vi "Abstract LV Class - Hierarchy.vi"   [LabVIEW 2021]
uses:
  Type/Abs_Type.lvclass
  Value/Abs_Value.lvclass
  Numeric/Abs_Numeric.lvclass
  Floating Point/Abs_Floating Point.lvclass
  Single Float/Abs_Single Float.lvclass
  Double Float/Abs_Double Float.lvclass
  Extended Float/Abs_Extended Float.lvclass
  Complex Double Float/Abs_Complex Double Float.lvclass
  Complex Extended Float/Abs_Complex Extended Float.lvclass
  Complex Single Float/Abs_Complex Single Float.lvclass
  Integer/Abs_Integer.lvclass
  I8 Integer/Abs_I8 Integer.lvclass
  I16 Integer/Abs_I16 Integer.lvclass
  I32 Integer/Abs_I32 Integer.lvclass
  I64 Integer/Abs_I64 Integer.lvclass
  U8 Integer/Abs_U8 Integer.lvclass
  U16 Integer/Abs_U16 Integer.lvclass
  U32 Integer/Abs_U32 Integer.lvclass
  U64 Integer/Abs_U64 Integer.lvclass
  Time/Abs_Time.lvclass
  Boolean/Abs_Boolean.lvclass
  String/Abs_String.lvclass
  Variant/Abs_Variant.lvclass
  Waveform/Abs_Waveform.lvclass
  Boolean/Static Write.vi
  Double Float/Simple Read.vi
  Boolean/Static Read.vi
  Numeric 1D/Abs_Numeric_1D.lvclass
  Single Float 1D/Abs_Single Float 1D.lvclass
  Double Float 1D/Abs_Double Float 1D.lvclass
  Extended Float 1D/Abs_Extended Float 1D.lvclass
  Complex Double Float 1D/Abs_Complex Double Float 1D.lvclass
  Complex Extended Float 1D/Abs_Complex Extended Float 1D.lvclass
  Complex Single Float 1D/Abs_Complex Single Float 1D.lvclass
panel:
  # "SEE DIAGRAM\nFOR Hierarchy"
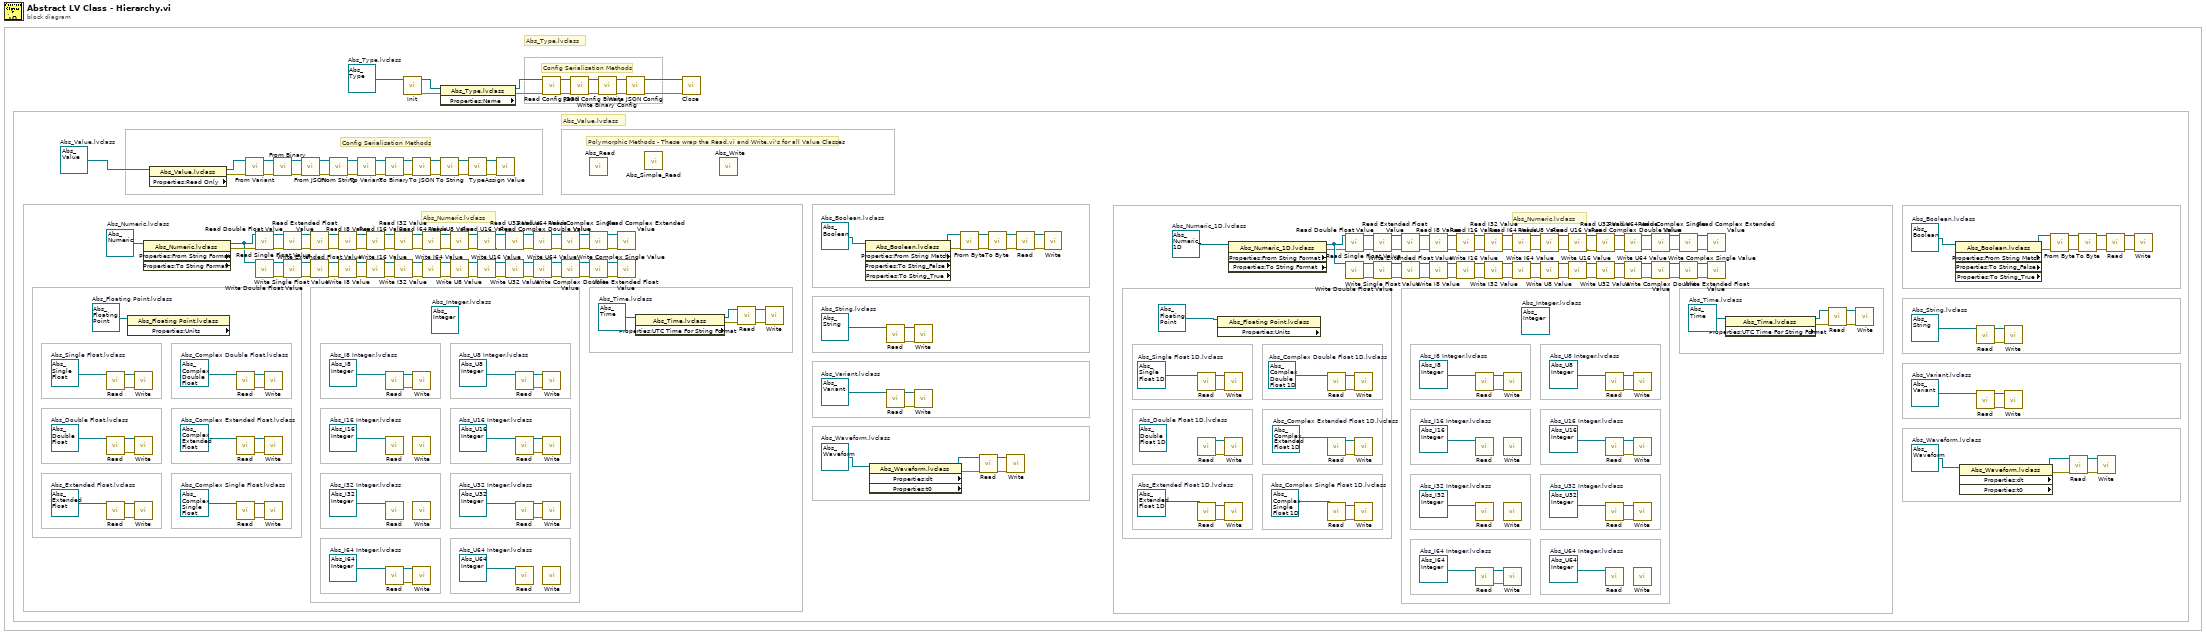
[diagram p0: block diagram]
diagram:
  w1 = refnum<class "Abs_Complex Single Float 1D.lvclass"> refnum  # Abs_Complex Single Float 1D.lvclass
  w2 = refnum<class "Abs_Complex Extended Float 1D.lvclass"> refnum  # Abs_Complex Extended Float 1D.lvclass
  w3 = refnum<class "Abs_Complex Double Float 1D.lvclass"> refnum  # Abs_Complex Double Float 1D.lvclass
  w4 = refnum<class "Abs_Extended Float 1D.lvclass"> refnum  # Abs_Extended Float 1D.lvclass
  (unwired) refnum<class "Abs_Double Float 1D.lvclass"> refnum  # Abs_Double Float 1D.lvclass
  w6 = refnum<class "Abs_Single Float 1D.lvclass"> refnum  # Abs_Single Float 1D.lvclass
  w7 = refnum<class "Abs_Numeric_1D.lvclass"> refnum  # Abs_Numeric_1D.lvclass
  w86 = refnum<class "Abs_Waveform.lvclass"> refnum  # Abs_Waveform.lvclass
  w85 = refnum<class "Abs_Variant.lvclass"> refnum  # Abs_Variant.lvclass
  w80 = refnum<class "Abs_String.lvclass"> refnum  # Abs_String.lvclass
  w71 = refnum<class "Abs_Boolean.lvclass"> refnum  # Abs_Boolean.lvclass
  w66 = refnum<class "Abs_Time.lvclass"> refnum  # Abs_Time.lvclass
  w56 = refnum<class "Abs_U64 Integer.lvclass"> refnum  # Abs_U64 Integer.lvclass
  w57 = refnum<class "Abs_U32 Integer.lvclass"> refnum  # Abs_U32 Integer.lvclass
  w59 = refnum<class "Abs_U16 Integer.lvclass"> refnum  # Abs_U16 Integer.lvclass
  w58 = refnum<class "Abs_U8 Integer.lvclass"> refnum  # Abs_U8 Integer.lvclass
  w53 = refnum<class "Abs_I64 Integer.lvclass"> refnum  # Abs_I64 Integer.lvclass
  w54 = refnum<class "Abs_I32 Integer.lvclass"> refnum  # Abs_I32 Integer.lvclass
  w55 = refnum<class "Abs_I16 Integer.lvclass"> refnum  # Abs_I16 Integer.lvclass
  w48 = refnum<class "Abs_I8 Integer.lvclass"> refnum  # Abs_I8 Integer.lvclass
  (unwired) refnum<class "Abs_Integer.lvclass"> refnum  # Abs_Integer.lvclass
  w160 = refnum<class "Abs_Waveform.lvclass"> refnum  # Abs_Waveform.lvclass
  w161 = refnum<class "Abs_Variant.lvclass"> refnum  # Abs_Variant.lvclass
  w166 = refnum<class "Abs_String.lvclass"> refnum  # Abs_String.lvclass
  w175 = refnum<class "Abs_Boolean.lvclass"> refnum  # Abs_Boolean.lvclass
  w180 = refnum<class "Abs_Time.lvclass"> refnum  # Abs_Time.lvclass
  w190 = refnum<class "Abs_U64 Integer.lvclass"> refnum  # Abs_U64 Integer.lvclass
  w189 = refnum<class "Abs_U32 Integer.lvclass"> refnum  # Abs_U32 Integer.lvclass
  w187 = refnum<class "Abs_U16 Integer.lvclass"> refnum  # Abs_U16 Integer.lvclass
  w188 = refnum<class "Abs_U8 Integer.lvclass"> refnum  # Abs_U8 Integer.lvclass
  w193 = refnum<class "Abs_I64 Integer.lvclass"> refnum  # Abs_I64 Integer.lvclass
  w192 = refnum<class "Abs_I32 Integer.lvclass"> refnum  # Abs_I32 Integer.lvclass
  w191 = refnum<class "Abs_I16 Integer.lvclass"> refnum  # Abs_I16 Integer.lvclass
  w198 = refnum<class "Abs_I8 Integer.lvclass"> refnum  # Abs_I8 Integer.lvclass
  (unwired) refnum<class "Abs_Integer.lvclass"> refnum  # Abs_Integer.lvclass
  w201 = refnum<class "Abs_Complex Single Float.lvclass"> refnum  # Abs_Complex Single Float.lvclass
  w204 = refnum<class "Abs_Complex Extended Float.lvclass"> refnum  # Abs_Complex Extended Float.lvclass
  w207 = refnum<class "Abs_Complex Double Float.lvclass"> refnum  # Abs_Complex Double Float.lvclass
  w210 = refnum<class "Abs_Extended Float.lvclass"> refnum  # Abs_Extended Float.lvclass
  w213 = refnum<class "Abs_Double Float.lvclass"> refnum  # Abs_Double Float.lvclass
  w216 = refnum<class "Abs_Single Float.lvclass"> refnum  # Abs_Single Float.lvclass
  w217 = refnum<class "Abs_Floating Point.lvclass"> refnum  # Abs_Floating Point.lvclass
  w245 = refnum<class "Abs_Numeric.lvclass"> refnum  # Abs_Numeric.lvclass
  w155 = refnum<class "Abs_Value.lvclass"> refnum  # Abs_Value.lvclass
  w268 = refnum<class "Abs_Type.lvclass"> refnum  # Abs_Type.lvclass
  # "Abs_Numeric.lvclass"
  # "Abs_Numeric.lvclass"
  # "Polymorphic Methods - These wrap the Read.vi and Write.vi's for all Value Classes"
  # "Config Serialisation Methods"
  # "Abs_Value.lvclass"
  # "Abs_Type.lvclass"
  # "Config Serialisation Methods"
  n1 = call-dynamic "Read.vi"("Double Float.lvclass_340760 in"=w216) -> ("error out"=w214:errorcluster, "Double Float.lvclass_340760 out"=w215:refnum<class "Abs_Single Float.lvclass">)  [unwired: 8 in, 1 out]
  n2 = call-dynamic "Read.vi"("Double Float.lvclass_340760 in"=w213) -> ("error out"=w211:errorcluster, "Double Float.lvclass_340760 out"=w212:refnum<class "Abs_Double Float.lvclass">)  [unwired: 8 in, 1 out]
  n3 = call-dynamic "Read.vi"("Double Float.lvclass_340760 in"=w210) -> ("error out"=w208:errorcluster, "Double Float.lvclass_340760 out"=w209:refnum<class "Abs_Extended Float.lvclass">)  [unwired: 8 in, 1 out]
  n4 = property class="Abs_Floating Point.lvclass" props=["Properties:Units"](reference=w217) -> ()  [unwired: 1 in, 3 out]
  n5 = call-dynamic "Write.vi"("error in (no error)"=w214, "Double Float.lvclass_340760 in"=w215) -> ()  [unwired: 8 in, 2 out]
  n6 = call-dynamic "Write.vi"("error in (no error)"=w211, "Double Float.lvclass in"=w212) -> ()  [unwired: 8 in, 2 out]
  n7 = call-dynamic "Write.vi"("error in (no error)"=w208, "Double Float.lvclass_340760 in"=w209) -> ()  [unwired: 8 in, 2 out]
  n8 = property class="Abs_Numeric.lvclass" props=["Properties:From String Format", "Properties:To String Format"](reference=w245) -> (reference out=w146:refnum<class "Abs_Numeric.lvclass">, error out=w244:errorcluster)  [unwired: 1 in, 2 out]
  n9 = property class="Abs_Value.lvclass" props=["Properties:Read Only"](reference=w155) -> (reference out=w153:refnum<class "Abs_Value.lvclass">, error out=w154:errorcluster)  [unwired: 1 in, 1 out]
  n10 = call-dynamic "Read.vi"("Double Float.lvclass_340760 in"=w207) -> ("error out"=w205:errorcluster, "Double Float.lvclass_340760 out"=w206:refnum<class "Abs_Complex Double Float.lvclass">)  [unwired: 8 in, 1 out]
  n11 = call-dynamic "Read.vi"("Double Float.lvclass_340760 in"=w204) -> ("error out"=w202:errorcluster, "Double Float.lvclass_340760 out"=w203:refnum<class "Abs_Complex Extended Float.lvclass">)  [unwired: 8 in, 1 out]
  n12 = call-dynamic "Read.vi"("Double Float.lvclass_340760 in"=w201) -> ("error out"=w199:errorcluster, "Double Float.lvclass_340760 out"=w200:refnum<class "Abs_Complex Single Float.lvclass">)  [unwired: 8 in, 1 out]
  n13 = call-dynamic "From Variant.vi"("error in (no error)"=w154, "Abs_Value in"=w153) -> ("error out"=w151:errorcluster, "Abs_Value out"=w152:refnum<class "Abs_Value.lvclass">)  [unwired: 8 in]
  n14 = call-dynamic "Read Double Float Value.vi"("error in (no error)"=w244, "Numeric in"=w146) -> ("error out"=w234:errorcluster, "Numeric out"=w243:refnum<class "Abs_Numeric.lvclass">)  [unwired: 7 in, 1 out]
  n15 = call-dynamic "Write Double Float Value.vi"("Numeric in"=w146) -> ("error out"=w132:errorcluster, "Numeric out"=w145:refnum<class "Abs_Numeric.lvclass">)  [unwired: 9 in]
  n16 = call-dynamic "Write.vi"("error in (no error)"=w205, "Double Float.lvclass_340760 in"=w206) -> ()  [unwired: 8 in, 2 out]
  n17 = call-dynamic "Write.vi"("error in (no error)"=w202, "Double Float.lvclass_340760 in"=w203) -> ()  [unwired: 8 in, 2 out]
  n18 = call-dynamic "Write.vi"("error in (no error)"=w199, "Double Float.lvclass_340760 in"=w200) -> ()  [unwired: 8 in, 2 out]
  n19 = call-dynamic "From Binary.vi"("error in (no error)"=w151, "Type in"=w152) -> ("error out"=w250:errorcluster, "Type out"=w255:refnum<class "Abs_Value.lvclass">)  [unwired: 7 in, 1 out]
  n20 = call-dynamic "Read Single Float Value.vi"("error in (no error)"=w234, "Numeric in"=w243) -> ("error out"=w233:errorcluster, "Numeric out"=w242:refnum<class "Abs_Numeric.lvclass">)  [unwired: 7 in, 1 out]
  n21 = call-dynamic "Write Single Float Value.vi"("error in (no error)"=w132, "Numeric in"=w145) -> ("error out"=w131:errorcluster, "Numeric out"=w144:refnum<class "Abs_Numeric.lvclass">)  [unwired: 8 in]
  n22 = call-dynamic "From JSON.vi"("error in (no error)"=w250, "Type in"=w255) -> ("error out"=w249:errorcluster, "Type out"=w254:refnum<class "Abs_Value.lvclass">)  [unwired: 8 in]
  n23 = call-dynamic "Read Extended Float Value.vi"("error in (no error)"=w233, "Numeric in"=w242) -> ("error out"=w232:errorcluster, "Numeric out"=w241:refnum<class "Abs_Numeric.lvclass">)  [unwired: 7 in, 1 out]
  n24 = call-dynamic "Write Extended Float Value.vi"("error in (no error)"=w131, "Numeric in"=w144) -> ("error out"=w130:errorcluster, "Numeric out"=w143:refnum<class "Abs_Numeric.lvclass">)  [unwired: 8 in]
  n25 = call-dynamic "From String.vi"("error in (no error)"=w249, "Type in"=w254) -> ("error out"=w149:errorcluster, "Type out"=w150:refnum<class "Abs_Value.lvclass">)  [unwired: 6 in, 2 out]
  n26 = call-dynamic "Read I8 Value.vi"("error in (no error)"=w232, "Numeric in"=w241) -> ("error out"=w231:errorcluster, "Numeric out"=w240:refnum<class "Abs_Numeric.lvclass">)  [unwired: 7 in, 1 out]
  n27 = call-dynamic "Write I8 Value.vi"("error in (no error)"=w130, "Numeric in"=w143) -> ("error out"=w129:errorcluster, "Numeric out"=w142:refnum<class "Abs_Numeric.lvclass">)  [unwired: 8 in]
  n28 = call-dynamic "To Variant.vi"("error in (no error)"=w149, "Abs_Value in"=w150) -> ("error out"=w147:errorcluster, "Abs_Value out"=w148:refnum<class "Abs_Value.lvclass">)  [unwired: 7 in, 1 out]
  n29 = call-dynamic "Read I16 Value.vi"("error in (no error)"=w231, "Numeric in"=w240) -> ("error out"=w230:errorcluster, "Numeric out"=w239:refnum<class "Abs_Numeric.lvclass">)  [unwired: 7 in, 1 out]
  n30 = call-dynamic "Write I16 Value.vi"("error in (no error)"=w129, "Numeric in"=w142) -> ("error out"=w128:errorcluster, "Numeric out"=w141:refnum<class "Abs_Numeric.lvclass">)  [unwired: 8 in]
  n31 = call-dynamic "To Binary.vi"("error in (no error)"=w147, "Type in"=w148) -> ("error out"=w248:errorcluster, "Type out"=w253:refnum<class "Abs_Value.lvclass">)  [unwired: 7 in, 1 out]
  n32 = call-dynamic "Read.vi"("Double Float.lvclass_340760 in"=w198) -> ("error out"=w196:errorcluster, "Double Float.lvclass_340760 out"=w197:refnum<class "Abs_I8 Integer.lvclass">)  [unwired: 8 in, 1 out]
  n33 = call-dynamic "Read.vi"("Double Float.lvclass_340760 in"=w191) -> ()  [unwired: 8 in, 3 out]
  n34 = call-dynamic "Read.vi"("Double Float.lvclass_340760 in"=w192) -> ()  [unwired: 8 in, 3 out]
  n35 = call-dynamic "Read.vi"("Double Float.lvclass_340760 in"=w193) -> ("error out"=w194:errorcluster, "Double Float.lvclass_340760 out"=w195:refnum<class "Abs_I64 Integer.lvclass">)  [unwired: 8 in, 1 out]
  n36 = call-dynamic "Read I32 Value.vi"("error in (no error)"=w230, "Numeric in"=w239) -> ("error out"=w229:errorcluster, "Numeric out"=w238:refnum<class "Abs_Numeric.lvclass">)  [unwired: 7 in, 1 out]
  n37 = call-dynamic "Write I32 Value.vi"("error in (no error)"=w128, "Numeric in"=w141) -> ("error out"=w127:errorcluster, "Numeric out"=w140:refnum<class "Abs_Numeric.lvclass">)  [unwired: 8 in]
  n38 = call-dynamic "Init.vi"("Data in"=w268) -> ("error out"=w267:errorcluster, "Data out"=w266:refnum<class "Abs_Type.lvclass">)  [unwired: 9 in]
  n39 = call-dynamic "To JSON.vi"("error in (no error)"=w248, "Type in"=w253) -> ("error out"=w247:errorcluster, "Type out"=w252:refnum<class "Abs_Value.lvclass">)  [unwired: 7 in, 1 out]
  n40 = call-dynamic "Write.vi"("error in (no error)"=w196, "Double Float.lvclass_340760 in"=w197) -> ()  [unwired: 8 in, 2 out]
  n41 = call-dynamic "Write.vi"() -> ()  [unwired: 10 in, 2 out]
  n42 = call-dynamic "Write.vi"() -> ()  [unwired: 10 in, 2 out]
  n43 = call-dynamic "Write.vi"("error in (no error)"=w194, "Double Float.lvclass_340760 in"=w195) -> ()  [unwired: 8 in, 2 out]
  n44 = call-dynamic "Read I64 Value.vi"("error in (no error)"=w229, "Numeric in"=w238) -> ("error out"=w228:errorcluster, "Numeric out"=w237:refnum<class "Abs_Numeric.lvclass">)  [unwired: 7 in, 1 out]
  n45 = call-dynamic "Write I64 Value.vi"("error in (no error)"=w127, "Numeric in"=w140) -> ("error out"=w126:errorcluster, "Numeric out"=w139:refnum<class "Abs_Numeric.lvclass">)  [unwired: 8 in]
  n46 = property class="Abs_Type.lvclass" props=["Properties:Name"](reference=w266, error in=w267) -> (reference out=w264:refnum<class "Abs_Type.lvclass">, error out=w265:errorcluster)  [unwired: 1 out]
  n47 = call-dynamic "To String.vi"("error in (no error)"=w247, "Types in"=w252) -> ("error out"=w246:errorcluster, "Types out"=w251:refnum<class "Abs_Value.lvclass">)  [unwired: 7 in, 1 out]
  n48 = call-dynamic "Read U8 Value.vi"("error in (no error)"=w228, "Numeric in"=w237) -> ("error out"=w227:errorcluster, "Numeric out"=w236:refnum<class "Abs_Numeric.lvclass">)  [unwired: 7 in, 1 out]
  n49 = call-dynamic "Write U8 Value.vi"("error in (no error)"=w126, "Numeric in"=w139) -> ("error out"=w125:errorcluster, "Numeric out"=w138:refnum<class "Abs_Numeric.lvclass">)  [unwired: 8 in]
  n50 = call-dynamic "Type.vi"("error in (no error)"=w246, "Element in"=w251) -> ("error out"=w118:errorcluster, "Element out"=w119:refnum<class "Abs_Value.lvclass">)  [unwired: 7 in, 1 out]
  n51 = call-dynamic "Read U16 Value.vi"("error in (no error)"=w227, "Numeric in"=w236) -> ("error out"=w226:errorcluster, "Numeric out"=w235:refnum<class "Abs_Numeric.lvclass">)  [unwired: 7 in, 1 out]
  n52 = call-dynamic "Write U16 Value.vi"("error in (no error)"=w125, "Numeric in"=w138) -> ("error out"=w124:errorcluster, "Numeric out"=w137:refnum<class "Abs_Numeric.lvclass">)  [unwired: 8 in]
  n53 = call-dynamic "Assign Value.vi"("error in (no error)"=w118, "Abs_Value in"=w119) -> ()  [unwired: 8 in, 2 out]
  n54 = call-dynamic "Read U32 Value.vi"("error in (no error)"=w226, "Numeric in"=w235) -> ("error out"=w225:errorcluster, "Numeric out"=w224:refnum<class "Abs_Numeric.lvclass">)  [unwired: 7 in, 1 out]
  n55 = call-dynamic "Write U32 Value.vi"("error in (no error)"=w124, "Numeric in"=w137) -> ("error out"=w123:errorcluster, "Numeric out"=w136:refnum<class "Abs_Numeric.lvclass">)  [unwired: 8 in]
  n56 = call-dynamic "Read.vi"("Double Float.lvclass_340760 in"=w188) -> ("error out"=w185:errorcluster, "Double Float.lvclass_340760 out"=w186:refnum<class "Abs_U8 Integer.lvclass">)  [unwired: 8 in, 1 out]
  n57 = call-dynamic "Read.vi"("Double Float.lvclass_340760 in"=w187) -> ("error out"=w183:errorcluster, "Double Float.lvclass_340760 out"=w184:refnum<class "Abs_U16 Integer.lvclass">)  [unwired: 8 in, 1 out]
  n58 = call-dynamic "Read.vi"("Double Float.lvclass_340760 in"=w189) -> ("error out"=w181:errorcluster, "Double Float.lvclass_340760 out"=w182:refnum<class "Abs_U32 Integer.lvclass">)  [unwired: 8 in, 1 out]
  n59 = call-dynamic "Read.vi"("Double Float.lvclass_340760 in"=w190) -> ()  [unwired: 8 in, 3 out]
  n60 = call-dynamic "Read U64 Value.vi"("error in (no error)"=w225, "Numeric in"=w224) -> ("error out"=w222:errorcluster, "Numeric out"=w223:refnum<class "Abs_Numeric.lvclass">)  [unwired: 7 in, 1 out]
  n61 = call-dynamic "Write U64 Value.vi"("error in (no error)"=w123, "Numeric in"=w136) -> ("error out"=w122:errorcluster, "Numeric out"=w135:refnum<class "Abs_Numeric.lvclass">)  [unwired: 8 in]
  n62 = call "Read Config JSON.vi"("error in (no error)"=w265, "Abs_Type in"=w264) -> ("error out"=w263:errorcluster, "Abs_Type out"=w262:refnum<class "Abs_Type.lvclass">)  [unwired: 8 in]
  n63 = call-dynamic "Write.vi"("error in (no error)"=w185, "Double Float.lvclass_340760 in"=w186) -> ()  [unwired: 8 in, 2 out]
  n64 = call-dynamic "Write.vi"("error in (no error)"=w183, "Double Float.lvclass_340760 in"=w184) -> ()  [unwired: 8 in, 2 out]
  n65 = call-dynamic "Write.vi"("error in (no error)"=w181, "Double Float.lvclass_340760 in"=w182) -> ()  [unwired: 8 in, 2 out]
  n66 = call-dynamic "Write.vi"() -> ()  [unwired: 10 in, 2 out]
  n67 = call-dynamic "Read Complex Double Value.vi"("error in (no error)"=w222, "Numeric in"=w223) -> ("error out"=w221:errorcluster, "Numeric out"=w220:refnum<class "Abs_Numeric.lvclass">)  [unwired: 7 in, 1 out]
  n68 = call-dynamic "Write Complex Double Value.vi"("error in (no error)"=w122, "Numeric in"=w135) -> ("error out"=w121:errorcluster, "Numeric out"=w134:refnum<class "Abs_Numeric.lvclass">)  [unwired: 8 in]
  n69 = call "Read Config Binary.vi"("error in (no error)"=w263, "Abs_Type in"=w262) -> ("error out"=w261:errorcluster, "Abs_Type out"=w260:refnum<class "Abs_Type.lvclass">)  [unwired: 7 in, 1 out]
  n70 = call-poly "Abs_Read.vi"() -> ()  [unwired: 9 in, 3 out]
  n71 = call-dynamic "Read Complex Single Value.vi"("error in (no error)"=w221, "Numeric in"=w220) -> ("error out"=w218:errorcluster, "Numeric out"=w219:refnum<class "Abs_Numeric.lvclass">)  [unwired: 7 in, 1 out]
  n72 = call-dynamic "Write Complex Single Value.vi"("error in (no error)"=w121, "Numeric in"=w134) -> ("error out"=w120:errorcluster, "Numeric out"=w133:refnum<class "Abs_Numeric.lvclass">)  [unwired: 8 in]
  n73 = call-dynamic "Write Binary Config.vi"("error in (no error)"=w261, "Abs_Type in"=w260) -> ("error out"=w258:errorcluster, "Abs_Type out"=w259:refnum<class "Abs_Type.lvclass">)  [unwired: 7 in, 1 out]
  n74 = call-dynamic "Read Complex Extended Value.vi"("error in (no error)"=w218, "Numeric in"=w219) -> ()  [unwired: 7 in, 3 out]
  n75 = call-dynamic "Write Extended Float Value.vi"("error in (no error)"=w120, "Numeric in"=w133) -> ()  [unwired: 8 in, 2 out]
  n76 = call-dynamic "Write JSON Config.vi"("error in (no error)"=w258, "Abs_Type in"=w259) -> ("error out"=w257:errorcluster, "Abs_Type out"=w256:refnum<class "Abs_Type.lvclass">)  [unwired: 7 in, 1 out]
  n77 = property class="Abs_Time.lvclass" props=["Properties:UTC Time For String Format"](reference=w180) -> (reference out=w176:refnum<class "Abs_Time.lvclass">, error out=w179:errorcluster)  [unwired: 1 in, 1 out]
  n78 = call-poly "Abs_Simple_Read.vi"() -> ()  [unwired: 5 in, 1 out]
  n79 = call-dynamic "Close.vi"("error in (no error)"=w257, "Data in"=w256) -> ()  [unwired: 8 in, 2 out]
  n80 = call-poly "Abs_Write.vi"() -> ()  [unwired: 10 in, 2 out]
  n81 = call-dynamic "Read.vi"("error in (no error)"=w179, "Double Float.lvclass_340760 in"=w176) -> ("error out"=w178:errorcluster, "Double Float.lvclass_340760 out"=w177:refnum<class "Abs_Time.lvclass">)  [unwired: 7 in, 1 out]
  n82 = call-dynamic "Write.vi"("error in (no error)"=w178, "Double Float.lvclass_340760 in"=w177) -> ()  [unwired: 8 in, 2 out]
  n83 = property class="Abs_Boolean.lvclass" props=["Properties:From String Match", "Properties:To String_False", "Properties:To String_True"](reference=w175) -> (reference out=w173:refnum<class "Abs_Boolean.lvclass">, error out=w174:errorcluster)  [unwired: 1 in, 3 out]
  n84 = property class="Abs_Waveform.lvclass" props=["Properties:dt", "Properties:t0"](reference=w160) -> (reference out=w159:refnum<class "Abs_Waveform.lvclass">, error out=w158:errorcluster)  [unwired: 1 in, 2 out]
  n85 = call-dynamic "Read.vi"("Abs_String in"=w166) -> ("error out"=w164:errorcluster, "Abs_String out"=w165:refnum<class "Abs_String.lvclass">)  [unwired: 8 in, 1 out]
  n86 = call-dynamic "Read.vi"("Abs_Variant in"=w161) -> ("error out"=w162:errorcluster, "Abs_Variant out"=w163:refnum<class "Abs_Variant.lvclass">)  [unwired: 8 in, 1 out]
  n87 = call-dynamic "Write.vi"("error in (no error)"=w164, "Abs_String in"=w165) -> ()  [unwired: 8 in, 2 out]
  n88 = call-dynamic "Write.vi"("error in (no error)"=w162, "Abs_Variant in"=w163) -> ()  [unwired: 8 in, 2 out]
  n89 = call-dynamic "From Byte.vi"("error in (no error)"=w174, "Boolean in"=w173) -> ("error out"=w171:errorcluster, "Boolean out"=w172:refnum<class "Abs_Boolean.lvclass">)  [unwired: 8 in]
  n90 = call-dynamic "Read.vi"("error in (no error)"=w158, "Abs_Waveform in"=w159) -> ("error out"=w157:errorcluster, "Abs_Waveform out"=w156:refnum<class "Abs_Waveform.lvclass">)  [unwired: 7 in, 1 out]
  n91 = call-dynamic "To Byte.vi"("error in (no error)"=w171, "Boolean in"=w172) -> ("error out"=w169:errorcluster, "Boolean out"=w170:refnum<class "Abs_Boolean.lvclass">)  [unwired: 8 in]
  n92 = call-dynamic "Write.vi"("error in (no error)"=w157, "Abs_Waveform in"=w156) -> ()  [unwired: 8 in, 2 out]
  n93 = call-dynamic "Read.vi"("error in (no error)"=w169, "Boolean in"=w170) -> ("error out"=w167:errorcluster, "Boolean out"=w168:refnum<class "Abs_Boolean.lvclass">)  [unwired: 7 in, 1 out]
  n94 = call-dynamic "Write.vi"("error in (no error)"=w167, "Boolean in"=w168) -> ()  [unwired: 8 in, 2 out]
  n95 = call-dynamic "Read.vi"("Double Float.lvclass_340760 in"=w6) -> ("error out"=w36:errorcluster, "Double Float.lvclass_340760 out"=w35:refnum<class "Abs_Single Float.lvclass">)  [unwired: 8 in, 1 out]
  n96 = call-dynamic "Read.vi"() -> ("error out"=w39:errorcluster, "Double Float.lvclass_340760 out"=w38:refnum<class "Abs_Double Float.lvclass">, "Double Float.lvclass_340760 in"=w37:refnum<class "Abs_Double Float.lvclass">)  [unwired: 8 in, 1 out]
  n97 = call-dynamic "Read.vi"("Double Float.lvclass_340760 in"=w4) -> ("error out"=w41:errorcluster, "Double Float.lvclass_340760 out"=w40:refnum<class "Abs_Extended Float.lvclass">)  [unwired: 8 in, 1 out]
  n98 = property class="Abs_Floating Point.lvclass" props=["Properties:Units"](reference=refnum<class "Abs_Floating Point.lvclass"> refnum ("Abs_Floating Point.lvclass")) -> ()  [unwired: 1 in, 3 out]
  n99 = call-dynamic "Write.vi"("error in (no error)"=w36, "Double Float.lvclass_340760 in"=w35) -> ()  [unwired: 8 in, 2 out]
  n100 = call-dynamic "Write.vi"("error in (no error)"=w39, "Double Float.lvclass in"=w38) -> ()  [unwired: 8 in, 2 out]
  n101 = call-dynamic "Write.vi"("error in (no error)"=w41, "Double Float.lvclass_340760 in"=w40) -> ()  [unwired: 8 in, 2 out]
  n102 = property class="Abs_Numeric_1D.lvclass" props=["Properties:From String Format", "Properties:To String Format"](reference=w7) -> (reference out=w91:refnum<class "Abs_Numeric_1D.lvclass">, error out=w8:errorcluster)  [unwired: 1 in, 2 out]
  n103 = call-dynamic "Read.vi"("Double Float.lvclass_340760 in"=w3) -> ("error out"=w43:errorcluster, "Double Float.lvclass_340760 out"=w42:refnum<class "Abs_Complex Double Float.lvclass">)  [unwired: 8 in, 1 out]
  n104 = call-dynamic "Read.vi"("Double Float.lvclass_340760 in"=w2) -> ("error out"=w45:errorcluster, "Double Float.lvclass_340760 out"=w44:refnum<class "Abs_Complex Extended Float.lvclass">)  [unwired: 8 in, 1 out]
  n105 = call-dynamic "Read.vi"("Double Float.lvclass_340760 in"=w1) -> ("error out"=w47:errorcluster, "Double Float.lvclass_340760 out"=w46:refnum<class "Abs_Complex Single Float.lvclass">)  [unwired: 8 in, 1 out]
  n106 = call-dynamic "Read Double Float Value.vi"("error in (no error)"=w8, "Numeric in"=w91) -> ("error out"=w18:errorcluster, "Numeric out"=w9:refnum<class "Abs_Numeric.lvclass">)  [unwired: 7 in, 1 out]
  n107 = call-dynamic "Write Double Float Value.vi"("Numeric in"=w91) -> ("error out"=w105:errorcluster, "Numeric out"=w92:refnum<class "Abs_Numeric.lvclass">)  [unwired: 9 in]
  n108 = call-dynamic "Write.vi"("error in (no error)"=w43, "Double Float.lvclass_340760 in"=w42) -> ()  [unwired: 8 in, 2 out]
  n109 = call-dynamic "Write.vi"("error in (no error)"=w45, "Double Float.lvclass_340760 in"=w44) -> ()  [unwired: 8 in, 2 out]
  n110 = call-dynamic "Write.vi"("error in (no error)"=w47, "Double Float.lvclass_340760 in"=w46) -> ()  [unwired: 8 in, 2 out]
  n111 = call-dynamic "Read Single Float Value.vi"("error in (no error)"=w18, "Numeric in"=w9) -> ("error out"=w19:errorcluster, "Numeric out"=w10:refnum<class "Abs_Numeric.lvclass">)  [unwired: 7 in, 1 out]
  n112 = call-dynamic "Write Single Float Value.vi"("error in (no error)"=w105, "Numeric in"=w92) -> ("error out"=w106:errorcluster, "Numeric out"=w93:refnum<class "Abs_Numeric.lvclass">)  [unwired: 8 in]
  n113 = call-dynamic "Read Extended Float Value.vi"("error in (no error)"=w19, "Numeric in"=w10) -> ("error out"=w20:errorcluster, "Numeric out"=w11:refnum<class "Abs_Numeric.lvclass">)  [unwired: 7 in, 1 out]
  n114 = call-dynamic "Write Extended Float Value.vi"("error in (no error)"=w106, "Numeric in"=w93) -> ("error out"=w107:errorcluster, "Numeric out"=w94:refnum<class "Abs_Numeric.lvclass">)  [unwired: 8 in]
  n115 = call-dynamic "Read I8 Value.vi"("error in (no error)"=w20, "Numeric in"=w11) -> ("error out"=w21:errorcluster, "Numeric out"=w12:refnum<class "Abs_Numeric.lvclass">)  [unwired: 7 in, 1 out]
  n116 = call-dynamic "Write I8 Value.vi"("error in (no error)"=w107, "Numeric in"=w94) -> ("error out"=w108:errorcluster, "Numeric out"=w95:refnum<class "Abs_Numeric.lvclass">)  [unwired: 8 in]
  n117 = call-dynamic "Read I16 Value.vi"("error in (no error)"=w21, "Numeric in"=w12) -> ("error out"=w22:errorcluster, "Numeric out"=w13:refnum<class "Abs_Numeric.lvclass">)  [unwired: 7 in, 1 out]
  n118 = call-dynamic "Write I16 Value.vi"("error in (no error)"=w108, "Numeric in"=w95) -> ("error out"=w109:errorcluster, "Numeric out"=w96:refnum<class "Abs_Numeric.lvclass">)  [unwired: 8 in]
  n119 = call-dynamic "Read.vi"("Double Float.lvclass_340760 in"=w48) -> ("error out"=w50:errorcluster, "Double Float.lvclass_340760 out"=w49:refnum<class "Abs_I8 Integer.lvclass">)  [unwired: 8 in, 1 out]
  n120 = call-dynamic "Read.vi"("Double Float.lvclass_340760 in"=w55) -> ()  [unwired: 8 in, 3 out]
  n121 = call-dynamic "Read.vi"("Double Float.lvclass_340760 in"=w54) -> ()  [unwired: 8 in, 3 out]
  n122 = call-dynamic "Read.vi"("Double Float.lvclass_340760 in"=w53) -> ("error out"=w52:errorcluster, "Double Float.lvclass_340760 out"=w51:refnum<class "Abs_I64 Integer.lvclass">)  [unwired: 8 in, 1 out]
  n123 = call-dynamic "Read I32 Value.vi"("error in (no error)"=w22, "Numeric in"=w13) -> ("error out"=w23:errorcluster, "Numeric out"=w14:refnum<class "Abs_Numeric.lvclass">)  [unwired: 7 in, 1 out]
  n124 = call-dynamic "Write I32 Value.vi"("error in (no error)"=w109, "Numeric in"=w96) -> ("error out"=w110:errorcluster, "Numeric out"=w97:refnum<class "Abs_Numeric.lvclass">)  [unwired: 8 in]
  n125 = call-dynamic "Write.vi"("error in (no error)"=w50, "Double Float.lvclass_340760 in"=w49) -> ()  [unwired: 8 in, 2 out]
  n126 = call-dynamic "Write.vi"() -> ()  [unwired: 10 in, 2 out]
  n127 = call-dynamic "Write.vi"() -> ()  [unwired: 10 in, 2 out]
  n128 = call-dynamic "Write.vi"("error in (no error)"=w52, "Double Float.lvclass_340760 in"=w51) -> ()  [unwired: 8 in, 2 out]
  n129 = call-dynamic "Read I64 Value.vi"("error in (no error)"=w23, "Numeric in"=w14) -> ("error out"=w24:errorcluster, "Numeric out"=w15:refnum<class "Abs_Numeric.lvclass">)  [unwired: 7 in, 1 out]
  n130 = call-dynamic "Write I64 Value.vi"("error in (no error)"=w110, "Numeric in"=w97) -> ("error out"=w111:errorcluster, "Numeric out"=w98:refnum<class "Abs_Numeric.lvclass">)  [unwired: 8 in]
  n131 = call-dynamic "Read U8 Value.vi"("error in (no error)"=w24, "Numeric in"=w15) -> ("error out"=w25:errorcluster, "Numeric out"=w16:refnum<class "Abs_Numeric.lvclass">)  [unwired: 7 in, 1 out]
  n132 = call-dynamic "Write U8 Value.vi"("error in (no error)"=w111, "Numeric in"=w98) -> ("error out"=w112:errorcluster, "Numeric out"=w99:refnum<class "Abs_Numeric.lvclass">)  [unwired: 8 in]
  n133 = call-dynamic "Read U16 Value.vi"("error in (no error)"=w25, "Numeric in"=w16) -> ("error out"=w26:errorcluster, "Numeric out"=w17:refnum<class "Abs_Numeric.lvclass">)  [unwired: 7 in, 1 out]
  n134 = call-dynamic "Write U16 Value.vi"("error in (no error)"=w112, "Numeric in"=w99) -> ("error out"=w113:errorcluster, "Numeric out"=w100:refnum<class "Abs_Numeric.lvclass">)  [unwired: 8 in]
  n135 = call-dynamic "Read U32 Value.vi"("error in (no error)"=w26, "Numeric in"=w17) -> ("error out"=w27:errorcluster, "Numeric out"=w28:refnum<class "Abs_Numeric.lvclass">)  [unwired: 7 in, 1 out]
  n136 = call-dynamic "Write U32 Value.vi"("error in (no error)"=w113, "Numeric in"=w100) -> ("error out"=w114:errorcluster, "Numeric out"=w101:refnum<class "Abs_Numeric.lvclass">)  [unwired: 8 in]
  n137 = call-dynamic "Read.vi"("Double Float.lvclass_340760 in"=w58) -> ("error out"=w61:errorcluster, "Double Float.lvclass_340760 out"=w60:refnum<class "Abs_U8 Integer.lvclass">)  [unwired: 8 in, 1 out]
  n138 = call-dynamic "Read.vi"("Double Float.lvclass_340760 in"=w59) -> ("error out"=w63:errorcluster, "Double Float.lvclass_340760 out"=w62:refnum<class "Abs_U16 Integer.lvclass">)  [unwired: 8 in, 1 out]
  n139 = call-dynamic "Read.vi"("Double Float.lvclass_340760 in"=w57) -> ("error out"=w65:errorcluster, "Double Float.lvclass_340760 out"=w64:refnum<class "Abs_U32 Integer.lvclass">)  [unwired: 8 in, 1 out]
  n140 = call-dynamic "Read.vi"("Double Float.lvclass_340760 in"=w56) -> ()  [unwired: 8 in, 3 out]
  n141 = call-dynamic "Read U64 Value.vi"("error in (no error)"=w27, "Numeric in"=w28) -> ("error out"=w30:errorcluster, "Numeric out"=w29:refnum<class "Abs_Numeric.lvclass">)  [unwired: 7 in, 1 out]
  n142 = call-dynamic "Write U64 Value.vi"("error in (no error)"=w114, "Numeric in"=w101) -> ("error out"=w115:errorcluster, "Numeric out"=w102:refnum<class "Abs_Numeric.lvclass">)  [unwired: 8 in]
  n143 = call-dynamic "Write.vi"("error in (no error)"=w61, "Double Float.lvclass_340760 in"=w60) -> ()  [unwired: 8 in, 2 out]
  n144 = call-dynamic "Write.vi"("error in (no error)"=w63, "Double Float.lvclass_340760 in"=w62) -> ()  [unwired: 8 in, 2 out]
  n145 = call-dynamic "Write.vi"("error in (no error)"=w65, "Double Float.lvclass_340760 in"=w64) -> ()  [unwired: 8 in, 2 out]
  n146 = call-dynamic "Write.vi"() -> ()  [unwired: 10 in, 2 out]
  n147 = call-dynamic "Read Complex Double Value.vi"("error in (no error)"=w30, "Numeric in"=w29) -> ("error out"=w31:errorcluster, "Numeric out"=w32:refnum<class "Abs_Numeric.lvclass">)  [unwired: 7 in, 1 out]
  n148 = call-dynamic "Write Complex Double Value.vi"("error in (no error)"=w115, "Numeric in"=w102) -> ("error out"=w116:errorcluster, "Numeric out"=w103:refnum<class "Abs_Numeric.lvclass">)  [unwired: 8 in]
  n149 = call-dynamic "Read Complex Single Value.vi"("error in (no error)"=w31, "Numeric in"=w32) -> ("error out"=w34:errorcluster, "Numeric out"=w33:refnum<class "Abs_Numeric.lvclass">)  [unwired: 7 in, 1 out]
  n150 = call-dynamic "Write Complex Single Value.vi"("error in (no error)"=w116, "Numeric in"=w103) -> ("error out"=w117:errorcluster, "Numeric out"=w104:refnum<class "Abs_Numeric.lvclass">)  [unwired: 8 in]
  n151 = call-dynamic "Read Complex Extended Value.vi"("error in (no error)"=w34, "Numeric in"=w33) -> ()  [unwired: 7 in, 3 out]
  n152 = call-dynamic "Write Extended Float Value.vi"("error in (no error)"=w117, "Numeric in"=w104) -> ()  [unwired: 8 in, 2 out]
  n153 = property class="Abs_Time.lvclass" props=["Properties:UTC Time For String Format"](reference=w66) -> (reference out=w70:refnum<class "Abs_Time.lvclass">, error out=w67:errorcluster)  [unwired: 1 in, 1 out]
  n154 = call-dynamic "Read.vi"("error in (no error)"=w67, "Double Float.lvclass_340760 in"=w70) -> ("error out"=w68:errorcluster, "Double Float.lvclass_340760 out"=w69:refnum<class "Abs_Time.lvclass">)  [unwired: 7 in, 1 out]
  n155 = call-dynamic "Write.vi"("error in (no error)"=w68, "Double Float.lvclass_340760 in"=w69) -> ()  [unwired: 8 in, 2 out]
  n156 = property class="Abs_Boolean.lvclass" props=["Properties:From String Match", "Properties:To String_False", "Properties:To String_True"](reference=w71) -> (reference out=w73:refnum<class "Abs_Boolean.lvclass">, error out=w72:errorcluster)  [unwired: 1 in, 3 out]
  n157 = property class="Abs_Waveform.lvclass" props=["Properties:dt", "Properties:t0"](reference=w86) -> (reference out=w87:refnum<class "Abs_Waveform.lvclass">, error out=w88:errorcluster)  [unwired: 1 in, 2 out]
  n158 = call-dynamic "Read.vi"("Abs_String in"=w80) -> ("error out"=w82:errorcluster, "Abs_String out"=w81:refnum<class "Abs_String.lvclass">)  [unwired: 8 in, 1 out]
  n159 = call-dynamic "Read.vi"("Abs_Variant in"=w85) -> ("error out"=w84:errorcluster, "Abs_Variant out"=w83:refnum<class "Abs_Variant.lvclass">)  [unwired: 8 in, 1 out]
  n160 = call-dynamic "Write.vi"("error in (no error)"=w82, "Abs_String in"=w81) -> ()  [unwired: 8 in, 2 out]
  n161 = call-dynamic "Write.vi"("error in (no error)"=w84, "Abs_Variant in"=w83) -> ()  [unwired: 8 in, 2 out]
  n162 = call-dynamic "From Byte.vi"("error in (no error)"=w72, "Boolean in"=w73) -> ("error out"=w75:errorcluster, "Boolean out"=w74:refnum<class "Abs_Boolean.lvclass">)  [unwired: 8 in]
  n163 = call-dynamic "Read.vi"("error in (no error)"=w88, "Abs_Waveform in"=w87) -> ("error out"=w89:errorcluster, "Abs_Waveform out"=w90:refnum<class "Abs_Waveform.lvclass">)  [unwired: 7 in, 1 out]
  n164 = call-dynamic "To Byte.vi"("error in (no error)"=w75, "Boolean in"=w74) -> ("error out"=w77:errorcluster, "Boolean out"=w76:refnum<class "Abs_Boolean.lvclass">)  [unwired: 8 in]
  n165 = call-dynamic "Write.vi"("error in (no error)"=w89, "Abs_Waveform in"=w90) -> ()  [unwired: 8 in, 2 out]
  n166 = call-dynamic "Read.vi"("error in (no error)"=w77, "Boolean in"=w76) -> ("error out"=w79:errorcluster, "Boolean out"=w78:refnum<class "Abs_Boolean.lvclass">)  [unwired: 7 in, 1 out]
  n167 = call-dynamic "Write.vi"("error in (no error)"=w79, "Boolean in"=w78) -> ()  [unwired: 8 in, 2 out]
